vi "set_temperature.vi"(3 "Temperature in":dbl) -> (0 "Pe0 out":dbl, 1 "Temperature out":dbl)   [LabVIEW 2015]
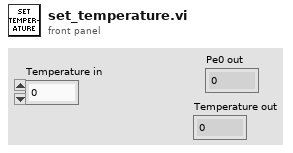
[diagram p1: front panel]
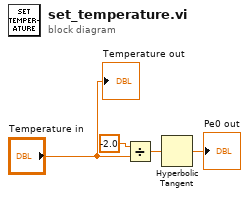
[diagram p0: block diagram]
diagram:
  n1 = Divide(x=-2.0, y="Temperature in") -> (x/y=w2:dbl)
  n2 = Hyperbolic Tangent(1:w2) -> (0:→"Pe0 out":dbl)
  "Temperature out" <- "Temperature in"
